vi "Set the Turn.vi"(8 "error in (no error)":errorcluster, 10 "Selector":dbl, 11 "Manejador de Turnos in":refnum<class "Manejador de Turnos.lvclass">) -> (0 "error out":errorcluster, 3 "Manejador de Turnos out":refnum<class "Manejador de Turnos.lvclass">)   [LabVIEW 2021, in "Manejador de Turnos.lvlib" / "Manejador de Turnos.lvclass"]
uses:
  Manejador de Turnos.lvclass
  Manejador de Turnos.lvclass/Manejador de Turnos.ctl
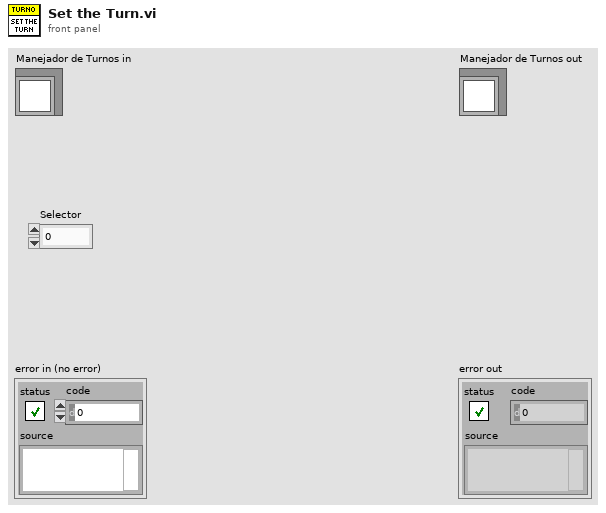
[diagram p1: front panel]
types:
  T1 = cluster{"Mojado":bool, "Enjabonado":bool, "Enjuagado":bool, "Secado":bool, "Aspirado":bool, "Lavado\nMotor":bool, "Encerado":bool}
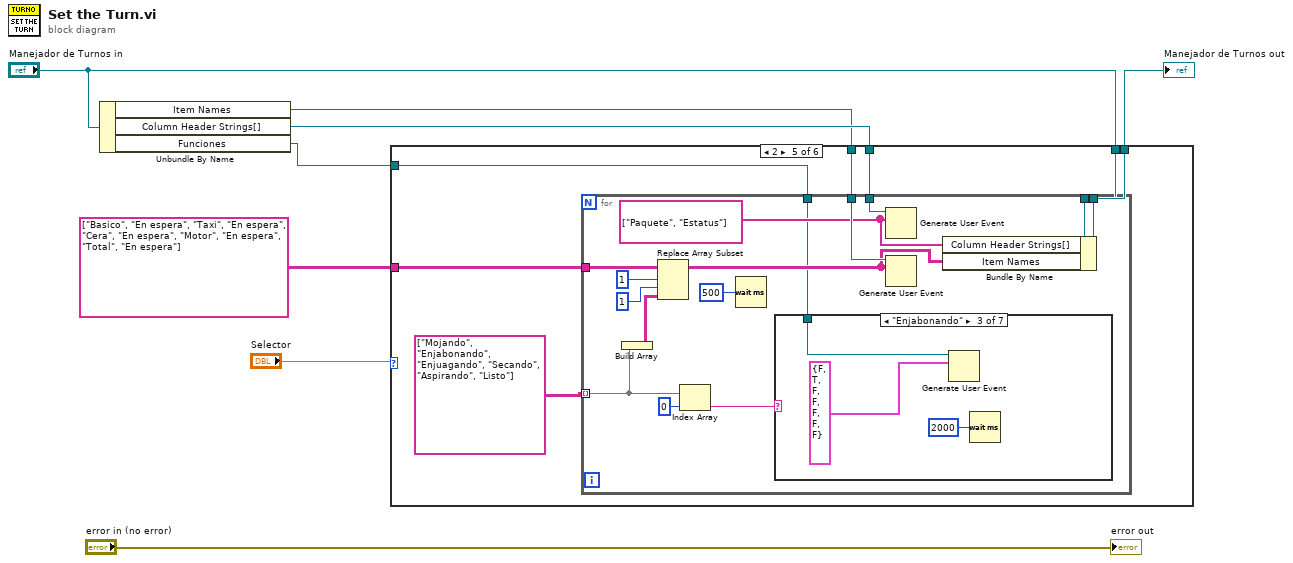
[diagram p0: block diagram]
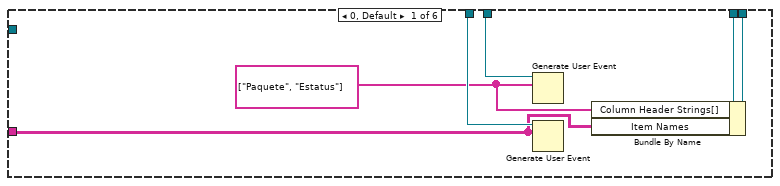
[diagram p2: hidden frame]
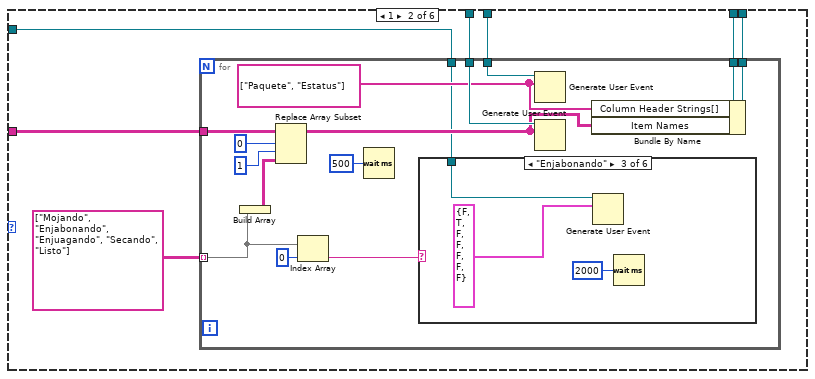
[diagram p3: hidden frame]
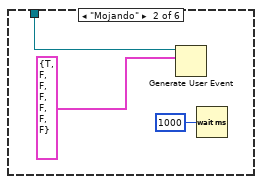
[diagram p5: hidden frame]
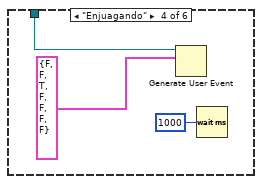
[diagram p6: hidden frame]
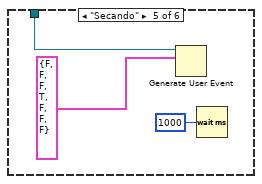
[diagram p7: hidden frame]
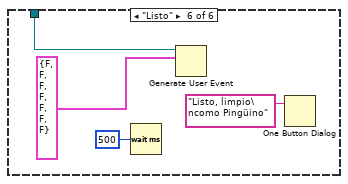
[diagram p8: hidden frame]
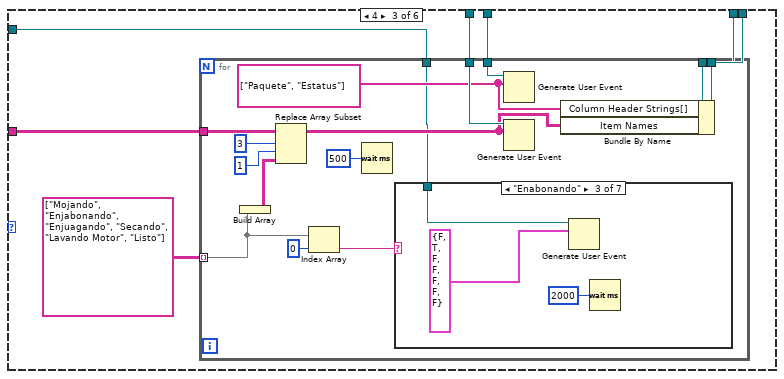
[diagram p9: hidden frame]
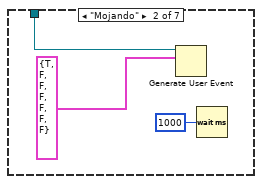
[diagram p11: hidden frame]
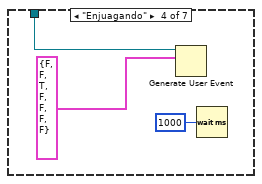
[diagram p12: hidden frame]
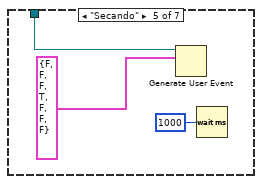
[diagram p13: hidden frame]
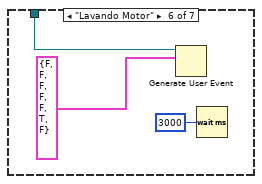
[diagram p14: hidden frame]
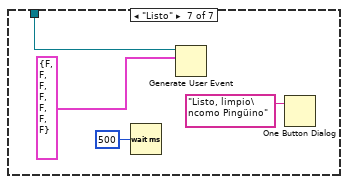
[diagram p15: hidden frame]
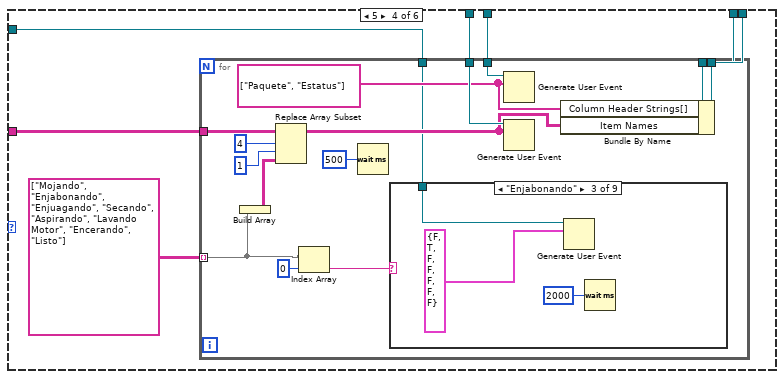
[diagram p16: hidden frame]
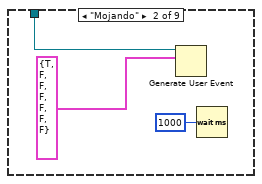
[diagram p18: hidden frame]
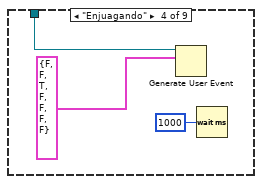
[diagram p19: hidden frame]
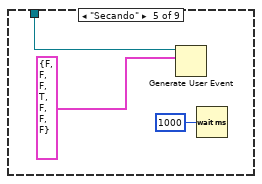
[diagram p20: hidden frame]
diagram:
  n1 = Unbundle By Name("Manejador de Turnos in") -> ("Item Names"=w5:refnum<user-event>, "Column Header Strings[]"=w6:refnum<user-event>, "Funciones"=w1:refnum<user-event>)
  n2 = case shown="2" "Selector" {
    tunnel: string[][] [["Basico", "En espera"], ["Taxi", "En espera"], ["Cera", "En espera"], ["Motor", "En espera"], ["Total", "En espera"]] ("Item Names") -> [w10 w21 w59 w100 w147 w188]
    tunnel: w6 -> [w14 w20 w58 w99 w146 w187]
    tunnel: w5 -> [w13 w19 w57 w98 w145 w186]
    tunnel: [w11 w18 w56 w97 w144 w185] -> w4
    tunnel: "Manejador de Turnos in" -> [w12 w17 w55 w96 w143 w184]
    tunnel: w1 -> [_ w15 w53 w94 w141 w182]
    frame 0, Default {
      w9 = string[] ["Paquete", "Estatus"] ("Row Header Strings[]")
      n3 = Generate User Event(user event=w14, event data cluster=w9) -> ()  [unwired: 2 in, 2 out]
      n4 = Generate User Event(user event=w13, event data cluster=w10) -> ()  [unwired: 2 in, 2 out]
      n5 = Bundle By Name(cluster=w12, "Column Header Strings[]"=w9, "Item Names"=w10) -> (w11:refnum<class "Manejador de Turnos.lvclass">)
    }
    frame 1 {
      n6 = for {
        tunnel: w21 -> [w35]
        tunnel: string[][] [["Mojando"], ["Enjabonando"], ["Enjuagando"], ["Secando"], ["Listo"]] -> [w25] mode=indexing
        tunnel: w20 -> [w32]
        tunnel: w19 -> [w31]
        tunnel: w17 -> [w30]
        tunnel: [w29] -> w18
        tunnel: w15 -> [w22]
        w28 = string[] ["Paquete", "Estatus"] ("Row Header Strings[]")
        n7 = Build Array(w25) -> (w26:string[][])
        n8 = Replace Array Subset(array=w35, new element=w26, index (row)=0 ("disabled index (row)"), index (col)=1 ("disabled index (row)")) -> (w27:string[][])
        n9 = Index Array(array=w25, index=0) -> (element=w23:string)
        n10 = Wait (ms)(milliseconds to wait=u32 500) -> ()  [unwired: 1 out]
        n11 = case shown="\"Enjabonando\"" w23 {
          tunnel: w22 -> [_ w39 w42 w45 w48 w52]
          frame " ", Default {
          }
          frame "Mojando" {
            n12 = Generate User Event(user event=w39, event data cluster=T1 {"Mojado"=TRUE, "Enjabonado"=FALSE, "Enjuagado"=FALSE, "Secado"=FALSE, "Aspirado"=FALSE, "Lavado\nMotor"=FALSE, "Encerado"=FALSE} ("event data")) -> ()  [unwired: 2 in, 2 out]
            n13 = Wait (ms)(milliseconds to wait=u32 1000) -> ()  [unwired: 1 out]
          }
          frame "Enjabonando" {
            n14 = Generate User Event(user event=w42, event data cluster=T1 {"Mojado"=FALSE, "Enjabonado"=TRUE, "Enjuagado"=FALSE, "Secado"=FALSE, "Aspirado"=FALSE, "Lavado\nMotor"=FALSE, "Encerado"=FALSE} ("event data")) -> ()  [unwired: 2 in, 2 out]
            n15 = Wait (ms)(milliseconds to wait=u32 2000) -> ()  [unwired: 1 out]
          }
          frame "Enjuagando" {
            n16 = Generate User Event(user event=w45, event data cluster=T1 {"Mojado"=FALSE, "Enjabonado"=FALSE, "Enjuagado"=TRUE, "Secado"=FALSE, "Aspirado"=FALSE, "Lavado\nMotor"=FALSE, "Encerado"=FALSE} ("event data")) -> ()  [unwired: 2 in, 2 out]
            n17 = Wait (ms)(milliseconds to wait=u32 1000) -> ()  [unwired: 1 out]
          }
          frame "Secando" {
            n18 = Generate User Event(user event=w48, event data cluster=T1 {"Mojado"=FALSE, "Enjabonado"=FALSE, "Enjuagado"=FALSE, "Secado"=TRUE, "Aspirado"=FALSE, "Lavado\nMotor"=FALSE, "Encerado"=FALSE} ("event data")) -> ()  [unwired: 2 in, 2 out]
            n19 = Wait (ms)(milliseconds to wait=u32 1000) -> ()  [unwired: 1 out]
          }
          frame "Listo" {
            n20 = Wait (ms)(milliseconds to wait=u32 500) -> ()  [unwired: 1 out]
            n21 = Generate User Event(user event=w52, event data cluster=T1 {"Mojado"=FALSE, "Enjabonado"=FALSE, "Enjuagado"=FALSE, "Secado"=FALSE, "Aspirado"=FALSE, "Lavado\nMotor"=FALSE, "Encerado"=FALSE} ("event data")) -> ()  [unwired: 2 in, 2 out]
            n22 = One Button Dialog(message="Listo, limpio\ncomo Pingüino") -> ()  [unwired: 1 in, 1 out]
          }
        }
        n23 = Generate User Event(user event=w32, event data cluster=w28) -> ()  [unwired: 2 in, 2 out]
        n24 = Generate User Event(user event=w31, event data cluster=w27) -> ()  [unwired: 2 in, 2 out]
        n25 = Bundle By Name(cluster=w30, "Column Header Strings[]"=w28, "Item Names"=w27) -> (w29:refnum<class "Manejador de Turnos.lvclass">)
      }
    }
    frame 4 {
      n26 = for {
        tunnel: w59 -> [w73]
        tunnel: string[][] [["Mojando"], ["Enjabonando"], ["Enjuagando"], ["Secando"], ["Lavando Motor"], ["Listo"]] -> [w62] mode=indexing
        tunnel: w58 -> [w69]
        tunnel: w57 -> [w68]
        tunnel: w55 -> [w67]
        tunnel: [w66] -> w56
        tunnel: w53 -> [w60]
        w65 = string[] ["Paquete", "Estatus"] ("Row Header Strings[]")
        n27 = Build Array(w62) -> (w70:string[][])
        n28 = Replace Array Subset(array=w73, new element=w70, index (row)=3 ("disabled index (row)"), index (col)=1 ("disabled index (row)")) -> (w64:string[][])
        n29 = Index Array(array=w62, index=0) -> (element=w61:string)
        n30 = Wait (ms)(milliseconds to wait=u32 500) -> ()  [unwired: 1 out]
        n31 = case shown="\"Enabonando\"" w61 {
          tunnel: w60 -> [_ w77 w80 w83 w86 w89 w93]
          frame " ", Default {
          }
          frame "Mojando" {
            n32 = Generate User Event(user event=w77, event data cluster=T1 {"Mojado"=TRUE, "Enjabonado"=FALSE, "Enjuagado"=FALSE, "Secado"=FALSE, "Aspirado"=FALSE, "Lavado\nMotor"=FALSE, "Encerado"=FALSE} ("event data")) -> ()  [unwired: 2 in, 2 out]
            n33 = Wait (ms)(milliseconds to wait=u32 1000) -> ()  [unwired: 1 out]
          }
          frame "Enabonando" {
            n34 = Generate User Event(user event=w80, event data cluster=T1 {"Mojado"=FALSE, "Enjabonado"=TRUE, "Enjuagado"=FALSE, "Secado"=FALSE, "Aspirado"=FALSE, "Lavado\nMotor"=FALSE, "Encerado"=FALSE} ("event data")) -> ()  [unwired: 2 in, 2 out]
            n35 = Wait (ms)(milliseconds to wait=u32 2000) -> ()  [unwired: 1 out]
          }
          frame "Enjuagando" {
            n36 = Generate User Event(user event=w83, event data cluster=T1 {"Mojado"=FALSE, "Enjabonado"=FALSE, "Enjuagado"=TRUE, "Secado"=FALSE, "Aspirado"=FALSE, "Lavado\nMotor"=FALSE, "Encerado"=FALSE} ("event data")) -> ()  [unwired: 2 in, 2 out]
            n37 = Wait (ms)(milliseconds to wait=u32 1000) -> ()  [unwired: 1 out]
          }
          frame "Secando" {
            n38 = Generate User Event(user event=w86, event data cluster=T1 {"Mojado"=FALSE, "Enjabonado"=FALSE, "Enjuagado"=FALSE, "Secado"=TRUE, "Aspirado"=FALSE, "Lavado\nMotor"=FALSE, "Encerado"=FALSE} ("event data")) -> ()  [unwired: 2 in, 2 out]
            n39 = Wait (ms)(milliseconds to wait=u32 1000) -> ()  [unwired: 1 out]
          }
          frame "Lavando Motor" {
            n40 = Generate User Event(user event=w89, event data cluster=T1 {"Mojado"=FALSE, "Enjabonado"=FALSE, "Enjuagado"=FALSE, "Secado"=FALSE, "Aspirado"=FALSE, "Lavado\nMotor"=TRUE, "Encerado"=FALSE} ("event data")) -> ()  [unwired: 2 in, 2 out]
            n41 = Wait (ms)(milliseconds to wait=u32 3000) -> ()  [unwired: 1 out]
          }
          frame "Listo" {
            n42 = Wait (ms)(milliseconds to wait=u32 500) -> ()  [unwired: 1 out]
            n43 = Generate User Event(user event=w93, event data cluster=T1 {"Mojado"=FALSE, "Enjabonado"=FALSE, "Enjuagado"=FALSE, "Secado"=FALSE, "Aspirado"=FALSE, "Lavado\nMotor"=FALSE, "Encerado"=FALSE} ("event data")) -> ()  [unwired: 2 in, 2 out]
            n44 = One Button Dialog(message="Listo, limpio\ncomo Pingüino") -> ()  [unwired: 1 in, 1 out]
          }
        }
        n45 = Generate User Event(user event=w69, event data cluster=w65) -> ()  [unwired: 2 in, 2 out]
        n46 = Generate User Event(user event=w68, event data cluster=w64) -> ()  [unwired: 2 in, 2 out]
        n47 = Bundle By Name(cluster=w67, "Column Header Strings[]"=w65, "Item Names"=w64) -> (w66:refnum<class "Manejador de Turnos.lvclass">)
      }
    }
    frame 5 {
      n48 = for {
        tunnel: w100 -> [w114]
        tunnel: string[][] [["Mojando"], ["Enjabonando"], ["Enjuagando"], ["Secando"], ["Aspirando"], ["Lavando Motor"], ["Encerando"], ["Listo"]] -> [w103] mode=indexing
        tunnel: w99 -> [w110]
        tunnel: w98 -> [w109]
        tunnel: w96 -> [w108]
        tunnel: [w107] -> w97
        tunnel: w94 -> [w101]
        w106 = string[] ["Paquete", "Estatus"] ("Row Header Strings[]")
        n49 = Build Array(w103) -> (w111:string[][])
        n50 = Replace Array Subset(array=w114, new element=w111, index (row)=4 ("disabled index (row)"), index (col)=1 ("disabled index (row)")) -> (w105:string[][])
        n51 = Index Array(array=w103, index=0) -> (element=w102:string)
        n52 = Wait (ms)(milliseconds to wait=u32 500) -> ()  [unwired: 1 out]
        n53 = case shown="\"Enjabonando\"" w102 {
          tunnel: w101 -> [_ w118 w121 w124 w127 w130 w133 w136 w140]
          frame " ", Default {
          }
          frame "Mojando" {
            n54 = Generate User Event(user event=w118, event data cluster=T1 {"Mojado"=TRUE, "Enjabonado"=FALSE, "Enjuagado"=FALSE, "Secado"=FALSE, "Aspirado"=FALSE, "Lavado\nMotor"=FALSE, "Encerado"=FALSE} ("event data")) -> ()  [unwired: 2 in, 2 out]
            n55 = Wait (ms)(milliseconds to wait=u32 1000) -> ()  [unwired: 1 out]
          }
          frame "Enjabonando" {
            n56 = Generate User Event(user event=w121, event data cluster=T1 {"Mojado"=FALSE, "Enjabonado"=TRUE, "Enjuagado"=FALSE, "Secado"=FALSE, "Aspirado"=FALSE, "Lavado\nMotor"=FALSE, "Encerado"=FALSE} ("event data")) -> ()  [unwired: 2 in, 2 out]
            n57 = Wait (ms)(milliseconds to wait=u32 2000) -> ()  [unwired: 1 out]
          }
          frame "Enjuagando" {
            n58 = Generate User Event(user event=w124, event data cluster=T1 {"Mojado"=FALSE, "Enjabonado"=FALSE, "Enjuagado"=TRUE, "Secado"=FALSE, "Aspirado"=FALSE, "Lavado\nMotor"=FALSE, "Encerado"=FALSE} ("event data")) -> ()  [unwired: 2 in, 2 out]
            n59 = Wait (ms)(milliseconds to wait=u32 1000) -> ()  [unwired: 1 out]
          }
          frame "Secando" {
            n60 = Generate User Event(user event=w127, event data cluster=T1 {"Mojado"=FALSE, "Enjabonado"=FALSE, "Enjuagado"=FALSE, "Secado"=TRUE, "Aspirado"=FALSE, "Lavado\nMotor"=FALSE, "Encerado"=FALSE} ("event data")) -> ()  [unwired: 2 in, 2 out]
            n61 = Wait (ms)(milliseconds to wait=u32 1000) -> ()  [unwired: 1 out]
          }
          frame "Aspirando" {
            n62 = Generate User Event(user event=w130, event data cluster=T1 {"Mojado"=FALSE, "Enjabonado"=FALSE, "Enjuagado"=FALSE, "Secado"=FALSE, "Aspirado"=TRUE, "Lavado\nMotor"=FALSE, "Encerado"=FALSE} ("event data")) -> ()  [unwired: 2 in, 2 out]
            n63 = Wait (ms)(milliseconds to wait=u32 2000) -> ()  [unwired: 1 out]
          }
          frame "Lavando Motor" {
            n64 = Generate User Event(user event=w133, event data cluster=T1 {"Mojado"=FALSE, "Enjabonado"=FALSE, "Enjuagado"=FALSE, "Secado"=FALSE, "Aspirado"=FALSE, "Lavado\nMotor"=TRUE, "Encerado"=FALSE} ("event data")) -> ()  [unwired: 2 in, 2 out]
            n65 = Wait (ms)(milliseconds to wait=u32 3000) -> ()  [unwired: 1 out]
          }
          frame "Encerando" {
            n66 = Generate User Event(user event=w136, event data cluster=T1 {"Mojado"=FALSE, "Enjabonado"=FALSE, "Enjuagado"=FALSE, "Secado"=FALSE, "Aspirado"=FALSE, "Lavado\nMotor"=FALSE, "Encerado"=TRUE} ("event data")) -> ()  [unwired: 2 in, 2 out]
            n67 = Wait (ms)(milliseconds to wait=u32 5000) -> ()  [unwired: 1 out]
          }
          frame "Listo" {
            n68 = Wait (ms)(milliseconds to wait=u32 500) -> ()  [unwired: 1 out]
            n69 = Generate User Event(user event=w140, event data cluster=T1 {"Mojado"=FALSE, "Enjabonado"=FALSE, "Enjuagado"=FALSE, "Secado"=FALSE, "Aspirado"=FALSE, "Lavado\nMotor"=FALSE, "Encerado"=FALSE} ("event data")) -> ()  [unwired: 2 in, 2 out]
            n70 = One Button Dialog(message="Listo, limpio\ncomo Pingüino") -> ()  [unwired: 1 in, 1 out]
          }
        }
        n71 = Generate User Event(user event=w110, event data cluster=w106) -> ()  [unwired: 2 in, 2 out]
        n72 = Generate User Event(user event=w109, event data cluster=w105) -> ()  [unwired: 2 in, 2 out]
        n73 = Bundle By Name(cluster=w108, "Column Header Strings[]"=w106, "Item Names"=w105) -> (w107:refnum<class "Manejador de Turnos.lvclass">)
      }
    }
    frame 2 {
      n74 = for {
        tunnel: w147 -> [w161]
        tunnel: string[][] [["Mojando"], ["Enjabonando"], ["Enjuagando"], ["Secando"], ["Aspirando"], ["Listo"]] -> [w150] mode=indexing
        tunnel: w146 -> [w157]
        tunnel: w145 -> [w156]
        tunnel: w143 -> [w155]
        tunnel: [w154] -> w144
        tunnel: w141 -> [w149]
        w153 = string[] ["Paquete", "Estatus"] ("Row Header Strings[]")
        n75 = Build Array(w150) -> (w158:string[][])
        n76 = Replace Array Subset(array=w161, new element=w158, index (row)=1 ("disabled index (row)"), index (col)=1 ("disabled index (row)")) -> (w152:string[][])
        n77 = Index Array(array=w150, index=0) -> (element=w148:string)
        n78 = Wait (ms)(milliseconds to wait=u32 500) -> ()  [unwired: 1 out]
        n79 = case shown="\"Enjabonando\"" w148 {
          tunnel: w149 -> [_ w165 w168 w171 w174 w177 w181]
          frame " ", Default {
          }
          frame "Mojando" {
            n80 = Generate User Event(user event=w165, event data cluster=T1 {"Mojado"=TRUE, "Enjabonado"=FALSE, "Enjuagado"=FALSE, "Secado"=FALSE, "Aspirado"=FALSE, "Lavado\nMotor"=FALSE, "Encerado"=FALSE} ("event data")) -> ()  [unwired: 2 in, 2 out]
            n81 = Wait (ms)(milliseconds to wait=u32 1000) -> ()  [unwired: 1 out]
          }
          frame "Enjabonando" {
            n82 = Generate User Event(user event=w168, event data cluster=T1 {"Mojado"=FALSE, "Enjabonado"=TRUE, "Enjuagado"=FALSE, "Secado"=FALSE, "Aspirado"=FALSE, "Lavado\nMotor"=FALSE, "Encerado"=FALSE} ("event data")) -> ()  [unwired: 2 in, 2 out]
            n83 = Wait (ms)(milliseconds to wait=u32 2000) -> ()  [unwired: 1 out]
          }
          frame "Enjuagando" {
            n84 = Generate User Event(user event=w171, event data cluster=T1 {"Mojado"=FALSE, "Enjabonado"=FALSE, "Enjuagado"=TRUE, "Secado"=FALSE, "Aspirado"=FALSE, "Lavado\nMotor"=FALSE, "Encerado"=FALSE} ("event data")) -> ()  [unwired: 2 in, 2 out]
            n85 = Wait (ms)(milliseconds to wait=u32 1000) -> ()  [unwired: 1 out]
          }
          frame "Secando" {
            n86 = Generate User Event(user event=w174, event data cluster=T1 {"Mojado"=FALSE, "Enjabonado"=FALSE, "Enjuagado"=FALSE, "Secado"=TRUE, "Aspirado"=FALSE, "Lavado\nMotor"=FALSE, "Encerado"=FALSE} ("event data")) -> ()  [unwired: 2 in, 2 out]
            n87 = Wait (ms)(milliseconds to wait=u32 1000) -> ()  [unwired: 1 out]
          }
          frame "Aspirando" {
            n88 = Generate User Event(user event=w177, event data cluster=T1 {"Mojado"=FALSE, "Enjabonado"=FALSE, "Enjuagado"=FALSE, "Secado"=FALSE, "Aspirado"=TRUE, "Lavado\nMotor"=FALSE, "Encerado"=FALSE} ("event data")) -> ()  [unwired: 2 in, 2 out]
            n89 = Wait (ms)(milliseconds to wait=u32 2000) -> ()  [unwired: 1 out]
          }
          frame "Listo" {
            n90 = Wait (ms)(milliseconds to wait=u32 500) -> ()  [unwired: 1 out]
            n91 = Generate User Event(user event=w181, event data cluster=T1 {"Mojado"=FALSE, "Enjabonado"=FALSE, "Enjuagado"=FALSE, "Secado"=FALSE, "Aspirado"=FALSE, "Lavado\nMotor"=FALSE, "Encerado"=FALSE} ("event data")) -> ()  [unwired: 2 in, 2 out]
            n92 = One Button Dialog(message="Listo, limpio\ncomo Pingüino") -> ()  [unwired: 1 in, 1 out]
          }
        }
        n93 = Generate User Event(user event=w157, event data cluster=w153) -> ()  [unwired: 2 in, 2 out]
        n94 = Generate User Event(user event=w156, event data cluster=w152) -> ()  [unwired: 2 in, 2 out]
        n95 = Bundle By Name(cluster=w155, "Column Header Strings[]"=w153, "Item Names"=w152) -> (w154:refnum<class "Manejador de Turnos.lvclass">)
      }
    }
    frame 3 {
      n96 = for {
        tunnel: w188 -> [w202]
        tunnel: string[][] [["Mojando"], ["Enjabonando"], ["Enjuagando"], ["Secando"], ["Aspirando"], ["Encerando"], ["Listo"]] -> [w190] mode=indexing
        tunnel: w187 -> [w198]
        tunnel: w186 -> [w197]
        tunnel: w184 -> [w196]
        tunnel: [w195] -> w185
        tunnel: w182 -> [w192]
        w194 = string[] ["Paquete", "Estatus"] ("Row Header Strings[]")
        n97 = Build Array(w190) -> (w199:string[][])
        n98 = Replace Array Subset(array=w202, new element=w199, index (row)=2 ("disabled index (row)"), index (col)=1 ("disabled index (row)")) -> (w193:string[][])
        n99 = Index Array(array=w190, index=0) -> (element=w189:string)
        n100 = Wait (ms)(milliseconds to wait=u32 500) -> ()  [unwired: 1 out]
        n101 = case shown="\"Enjabonando\"" w189 {
          tunnel: w192 -> [_ w206 w209 w212 w215 w218 w221 w225]
          frame " ", Default {
          }
          frame "Mojando" {
            n102 = Generate User Event(user event=w206, event data cluster=T1 {"Mojado"=TRUE, "Enjabonado"=FALSE, "Enjuagado"=FALSE, "Secado"=FALSE, "Aspirado"=FALSE, "Lavado\nMotor"=FALSE, "Encerado"=FALSE} ("event data")) -> ()  [unwired: 2 in, 2 out]
            n103 = Wait (ms)(milliseconds to wait=u32 1000) -> ()  [unwired: 1 out]
          }
          frame "Enjabonando" {
            n104 = Generate User Event(user event=w209, event data cluster=T1 {"Mojado"=FALSE, "Enjabonado"=TRUE, "Enjuagado"=FALSE, "Secado"=FALSE, "Aspirado"=FALSE, "Lavado\nMotor"=FALSE, "Encerado"=FALSE} ("event data")) -> ()  [unwired: 2 in, 2 out]
            n105 = Wait (ms)(milliseconds to wait=u32 2000) -> ()  [unwired: 1 out]
          }
          frame "Enjuagando" {
            n106 = Generate User Event(user event=w212, event data cluster=T1 {"Mojado"=FALSE, "Enjabonado"=FALSE, "Enjuagado"=TRUE, "Secado"=FALSE, "Aspirado"=FALSE, "Lavado\nMotor"=FALSE, "Encerado"=FALSE} ("event data")) -> ()  [unwired: 2 in, 2 out]
            n107 = Wait (ms)(milliseconds to wait=u32 1000) -> ()  [unwired: 1 out]
          }
          frame "Secando" {
            n108 = Generate User Event(user event=w215, event data cluster=T1 {"Mojado"=FALSE, "Enjabonado"=FALSE, "Enjuagado"=FALSE, "Secado"=TRUE, "Aspirado"=FALSE, "Lavado\nMotor"=FALSE, "Encerado"=FALSE} ("event data")) -> ()  [unwired: 2 in, 2 out]
            n109 = Wait (ms)(milliseconds to wait=u32 1000) -> ()  [unwired: 1 out]
          }
          frame "Aspirando" {
            n110 = Generate User Event(user event=w218, event data cluster=T1 {"Mojado"=FALSE, "Enjabonado"=FALSE, "Enjuagado"=FALSE, "Secado"=FALSE, "Aspirado"=TRUE, "Lavado\nMotor"=FALSE, "Encerado"=FALSE} ("event data")) -> ()  [unwired: 2 in, 2 out]
            n111 = Wait (ms)(milliseconds to wait=u32 2000) -> ()  [unwired: 1 out]
          }
          frame "Encerando" {
            n112 = Generate User Event(user event=w221, event data cluster=T1 {"Mojado"=FALSE, "Enjabonado"=FALSE, "Enjuagado"=FALSE, "Secado"=FALSE, "Aspirado"=FALSE, "Lavado\nMotor"=FALSE, "Encerado"=TRUE} ("event data")) -> ()  [unwired: 2 in, 2 out]
            n113 = Wait (ms)(milliseconds to wait=u32 5000) -> ()  [unwired: 1 out]
          }
          frame "Listo" {
            n114 = Wait (ms)(milliseconds to wait=u32 500) -> ()  [unwired: 1 out]
            n115 = Generate User Event(user event=w225, event data cluster=T1 {"Mojado"=FALSE, "Enjabonado"=FALSE, "Enjuagado"=FALSE, "Secado"=FALSE, "Aspirado"=FALSE, "Lavado\nMotor"=FALSE, "Encerado"=FALSE} ("event data")) -> ()  [unwired: 2 in, 2 out]
            n116 = One Button Dialog(message="Listo, limpio\ncomo Pingüino") -> ()  [unwired: 1 in, 1 out]
          }
        }
        n117 = Generate User Event(user event=w198, event data cluster=w194) -> ()  [unwired: 2 in, 2 out]
        n118 = Generate User Event(user event=w197, event data cluster=w193) -> ()  [unwired: 2 in, 2 out]
        n119 = Bundle By Name(cluster=w196, "Column Header Strings[]"=w194, "Item Names"=w193) -> (w195:refnum<class "Manejador de Turnos.lvclass">)
      }
    }
  }
  "Manejador de Turnos out" <- w4
  "error out" <- "error in (no error)"
